vi "BuildDecisionTree.vi"(8 "error in (no error)":errorcluster, 9 "Current Player":T1, 10 "Gameboard":T2, 11 "DecisionTree In":T3) -> (0 "error out":errorcluster, 2 "Status":T1, 3 "DecisionTree Out":T3)   [LabVIEW 2020]
uses:
  controls/DecisionTree.ctl
  controls/Gameboard Data.ctl
  controls/DecisionTreeRecord.ctl
  controls/Player.ctl
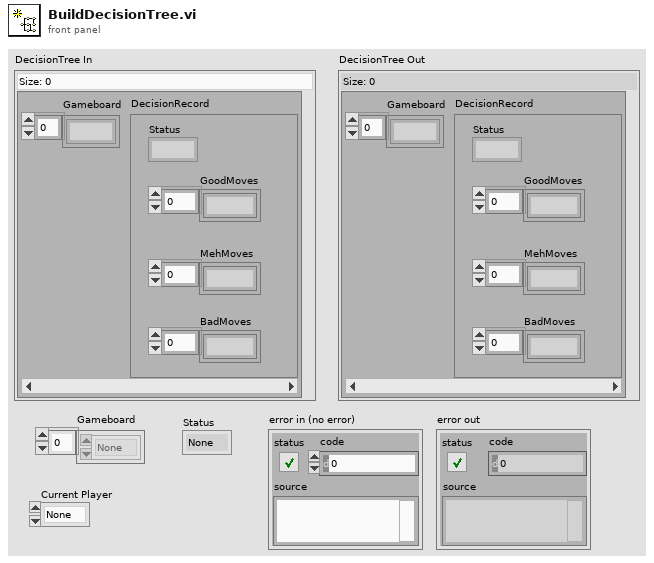
[diagram p1: front panel]
types:
  T1 = typedef "Player.ctl" = enum16{"None", "Player 1", "Player 2"}
  T2 = typedef "Gameboard Data.ctl" = enum16{"None", "Player 1", "Player 2"}[]
  T3 = typedef "DecisionTree.ctl" = map{T2, T4}
  T4 = typedef "DecisionTreeRecord.ctl" = cluster{"Status":T1, "GoodMoves":i8[], "MehMoves":i8[], "BadMoves":i8[]}
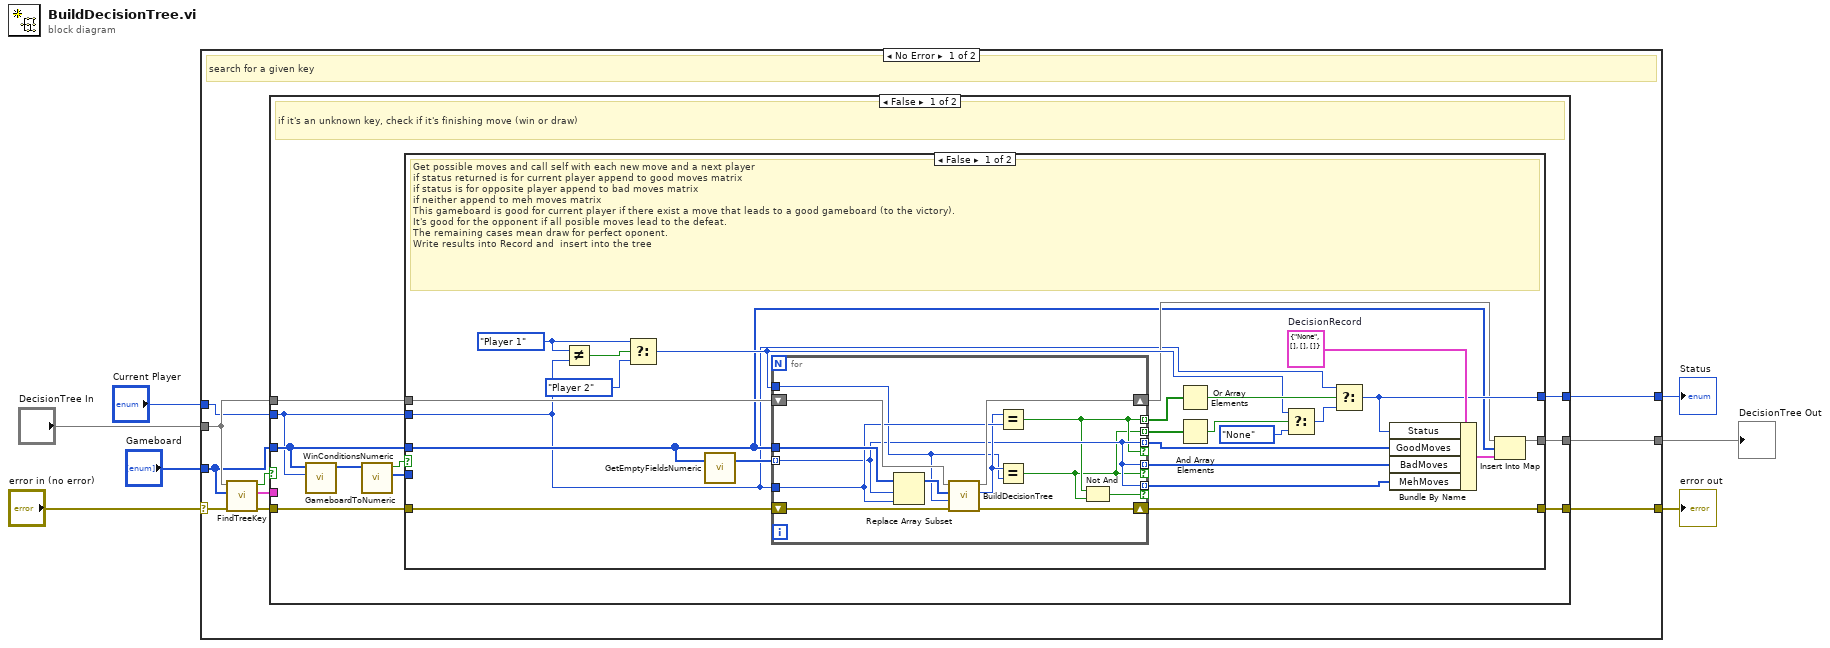
[diagram p0: block diagram]
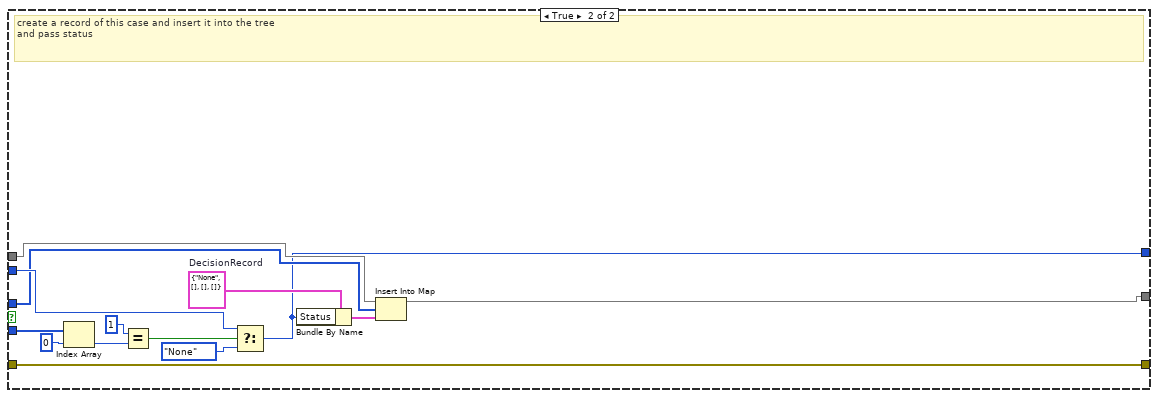
[diagram p2: hidden frame]
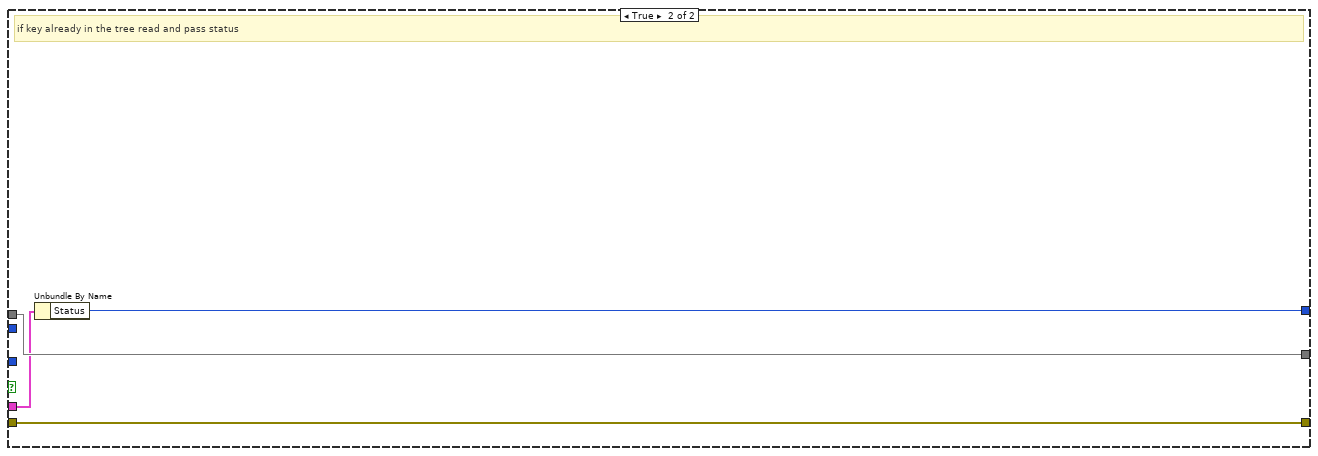
[diagram p3: hidden frame]
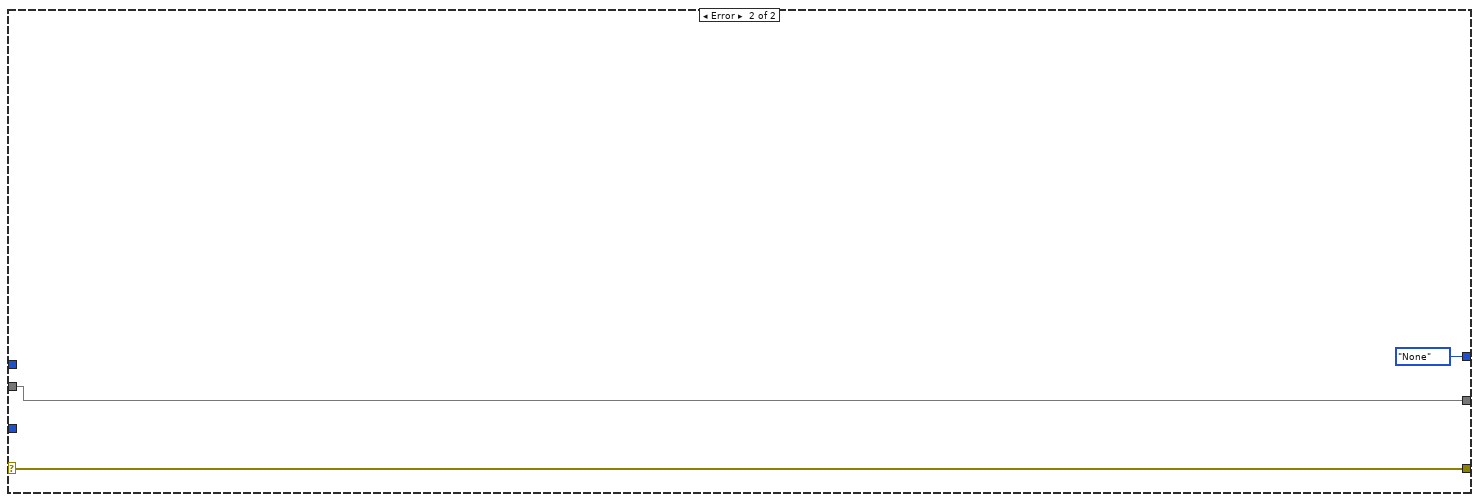
[diagram p4: hidden frame]
diagram:
  n1 = case shown="No Error" "error in (no error)" {
    selector: "error in (no error)" -> [w17 w85]
    tunnel: [w12 w85] -> w6
    tunnel: "Gameboard" -> [w9 _]
    tunnel: "Current Player" -> [w8 _]
    tunnel: [w10 Player."None" ("Status")] -> w3
    tunnel: "DecisionTree In" -> [w14 w83]
    tunnel: [w13 w83] -> w1
    frame No Error {
      # "search for a given key"
      n2 = call "FindTreeKey.vi"("error in (no error)"=w17, "Key"=w9, "Map"=w14) -> ("error out"=w15:errorcluster, "DecisionRecord"=w11:T4, "IsFound?"=w16:bool)  [unwired: 5 in, 1 out]
      n3 = case shown="False" w16 {
        tunnel: w15 -> [w22 w81]
        tunnel: w14 -> [w21 w82]
        tunnel: [w20 w82] -> w13
        tunnel: [w18 w81] -> w12
        tunnel: w11 -> [_ w80]
        tunnel: [w19 w79] -> w10
        tunnel: w9 -> [w24 _]
        tunnel: w8 -> [w23 _]
        frame False {
          # "if it's an unknown key, check if it's finishing move (win or draw)"
          n4 = call "GameboardToNumeric.vi"("CurrentPlayer"=w23, "Gameboard"=w24) -> ("NumericGameboard"=w25:i8[])  [unwired: 9 in]
          n5 = call "WinConditionsNumeric.vi"("NumericGameboard"=w25) -> ("LineIndices"=w26:i8[], "End?"=w27:bool)  [unwired: 9 in]
          n6 = case shown="False" w27 {
            tunnel: w26 -> [_ w78]
            tunnel: w24 -> [w31 w68]
            tunnel: w23 -> [w30 w73]
            tunnel: w22 -> [w48 w65]
            tunnel: w21 -> [w49 w70]
            tunnel: [w34 w69] -> w20
            tunnel: [w36 w66] -> w19
            tunnel: [w32 w65] -> w18
            frame False {
              w40 = T4 {"Status"=enum."None", "GoodMoves"=[], "MehMoves"=[], "BadMoves"=[]}  # DecisionRecord
              w29 = Player."Player 1" ("y")
              # "Get possible moves and call self with each new move and a next player\nif status returned is for current player append to good moves matrix\nif status is for opposite player append to bad moves matrix\nif neither append to meh moves matrix\nThis gameboard is good for current player if there exist a move that leads to a good gameboard (to the victory).\nIt's good for the opponent if all posible moves lead to the defeat. \nThe remaining cases mean draw for perfect oponent.\nWrite results into Record and  insert into the tree"
              n7 = Not Equal?(x=w29, y=w30) -> (x != y?=w50:bool)
              n8 = Select(t=w29, s=w50, f=Player."Player 2") -> (s? t:f=w42:T1)
              n9 = call "GetEmptyFieldsNumeric.vi"("NumericGameboard"=w31) -> ("Indices"=w51:i8[])  [unwired: 2 in]
              n10 = for {
                tunnel: w51 -> [w55] mode=indexing
                tunnel: w31 -> [w64]
                tunnel: w30 -> [w58]
                tunnel: w42 -> [w56]
                shift-right: [w60] -> w35
                shift-left: w49 -> [w63]
                shift-right: [w59] -> w32
                shift-left: w48 -> [w61]
                tunnel: [w55] -> w39 mode=indexing if=w53
                tunnel: [w55] -> w38 mode=indexing if=w52
                tunnel: [w55] -> w37 mode=indexing if=w54
                tunnel: [w53] -> w47 mode=indexing
                tunnel: [w52] -> w46 mode=indexing
                n11 = Replace Array Subset(array=w64, new element=w58, index=w55) -> (w62:T2)
                n12 = call "BuildDecisionTree.vi"("error in (no error)"=w61, "Current Player"=w56, "Gameboard"=w62, "DecisionTree In"=w63) -> ("error out"=w59:errorcluster, "Status"=w57:T1, "DecisionTree Out"=w60:T3)  [unwired: 5 in]
                n13 = Equal?(x=w57, y=w58) -> (x = y?=w53:bool)
                n14 = Equal?(x=w57, y=w56) -> (x = y?=w52:bool)
                n15 = Not And(1:w52, 2:w53) -> (0:w54:bool)
              }
              n16 = Or Array Elements(Boolean array=w47) -> (logical OR=w45:bool)
              n17 = And Array Elements(Boolean array=w46) -> (logical AND=w43:bool)
              n18 = Select(t=w42, s=w43, f=Player."None") -> (s? t:f=w44:T1)
              n19 = Select(t=w30, s=w45, f=w44) -> (s? t:f=w36:T1)
              n20 = Bundle By Name(cluster=w40, "Status"=w36, "GoodMoves"=w39, "BadMoves"=w38, "MehMoves"=w37) -> (w33:T4)
              n21 = Insert Into Map(map in=w35, key=w31, value=w33) -> (map out=w34:T3)  [unwired: 2 out]
            }
            frame True {
              w71 = T4 {"Status"=enum."None", "GoodMoves"=[], "MehMoves"=[], "BadMoves"=[]}  # DecisionRecord
              # "create a record of this case and insert it into the tree\nand pass status"
              n22 = Index Array(array=w78, index=0) -> (element=w76:i8)
              n23 = Equal?(x=i8 1, y=w76) -> (x = y?=w74:bool)
              n24 = Select(t=w73, s=w74, f=Player."None") -> (s? t:f=w66:T1)
              n25 = Bundle By Name(cluster=w71, "Status"=w66) -> (w67:T4)
              n26 = Insert Into Map(map in=w70, key=w68, value=w67) -> (map out=w69:T3)  [unwired: 2 out]
            }
          }
        }
        frame True {
          # "if key already in the tree read and pass status"
          n27 = Unbundle By Name(w80) -> ("Status"=w79:T1)
        }
      }
    }
    frame Error {
    }
  }
  "DecisionTree Out" <- w1
  "error out" <- w6
  "Status" <- w3
